vi "Get Distance between two points.vi"(11 "Array":dbl[](array[numeric])) -> (2 "Line ROI coordinates":T1 {"Start X" scale=0.0..1024.0; "End X" scale=0.0..1024.0}, 3 "appended array":dbl[](array[numeric]))   [LabVIEW 2020]
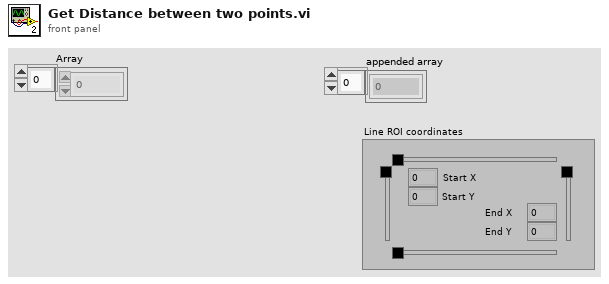
[diagram p1: front panel]
types:
  T1 = typedef "IMAQ Line" = cluster{"Start X":i32, "Start Y":i32, "End X":i32, "End Y":i32}
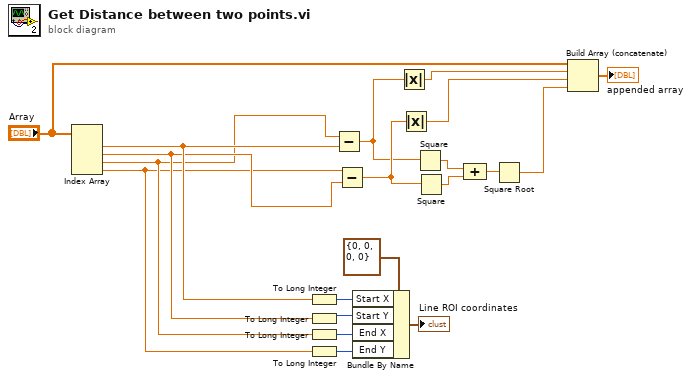
[diagram p0: block diagram]
diagram:
  n1 = Index Array(array="Array") -> (element #1=w5:dbl, element #2=w4:dbl, element #3=w3:dbl, element #4=w2:dbl)  [unwired: 4 in]
  n2 = To Long Integer(number=w5) -> (32bit integer=w9:i32)
  n3 = To Long Integer(number=w4) -> (32bit integer=w8:i32)
  n4 = To Long Integer(number=w3) -> (32bit integer=w6:i32)
  n5 = To Long Integer(number=w2) -> (32bit integer=w7:i32)
  n6 = Subtract(x=w3, y=w5) -> (x-y=w19:dbl)
  n7 = Subtract(x=w2, y=w4) -> (x-y=w20:dbl)
  n8 = Bundle By Name(cluster=T1 {"Start X"=0, "Start Y"=0, "End X"=0, "End Y"=0} ("Line"), "Start X"=w9, "Start Y"=w8, "End X"=w6, "End Y"=w7) -> (→"Line ROI coordinates":T1)
  n9 = Absolute Value(x=w19) -> (abs(x)=w14:dbl)
  n10 = Absolute Value(x=w20) -> (abs(x)=w13:dbl)
  n11 = Square(x=w19) -> (x^2=w17:dbl)
  n12 = Square(x=w20) -> (x^2=w16:dbl)
  n13 = Compound Arithmetic op=ADD(w17, w16) -> (w18:dbl)
  n14 = Square Root(x=w18) -> (sqrt(x)=w12:dbl)
  n15 = Build Array (concatenate)("Array", w14, w13, w12) -> (→"appended array":dbl[])
